vi "Main.vi"(11 "Module Admin":refnum<class "Delacor_lib_QMH_Module Admin.lvclass">) -> ()   [LabVIEW 2020, in "Settings.lvlib"]
doc: "This template is based off of the Queued Message Handler design pattern and the Queued Message Handler project template that ships with LabVIEW.\n\nThe main difference is that the queue is private to this module and communication between modules is performed via Broadcast and Request events.\n\nRequest events are wrapped in public API methods and are handled in the Event Handling Loop (EHL) of this VI. Any module can register for Broadcast events sent by this module. The EHL generates messages based on user interface actions.\n\nThe Message Handling Loop (MHL) processes messages generated by the EHL, or by other messages. The messages are string values, so new messages can be added easily to the Message Cases case structure in the MHL. Each message cluster can also provide an optional value for Message Data, which is a variant that can be converted to whatever message-specific data is required.\n_____\nBased on Delacor QMH Project Template 6.0.0.89."
uses:
  Settings.lvlib
  <vilib>/Delacor/Delacor QMH/Libraries/Module Admin_class/Delacor_lib_QMH_Module Admin.lvclass
  Acquisition/cluster analogico.ctl
  Acquisition/cluster digital.ctl
  Module Data--cluster.ctl
  Stop Argument--cluster.ctl
  <vilib>/Delacor/Delacor QMH/Libraries/Message Queue_class/Delacor_lib_QMH_Message Queue.lvclass/Delacor_lib_QMH_Message Queue.ctl
  <vilib>/Delacor/Delacor QMH/Libraries/Module Admin_class/Delacor_lib_QMH_Module Admin.lvclass/Delacor_lib_QMH_Module Admin.ctl
  ADD TASK Argument--cluster.ctl
  Erase all Argument--cluster.ctl
  <vilib>/Utility/miscctls.llb/LVPointTypeDef.ctl
  <vilib>/Delacor/Delacor QMH/Libraries/Message Queue_class/Delacor_lib_QMH_Enqueue Message (Single).vi
  <vilib>/Delacor/Delacor QMH/Libraries/Module Admin_class/Delacor_lib_QMH_Get External Launch.vi
  <vilib>/Utility/error.llb/Error Cluster From Error Code.vi
  <vilib>/ErrorRing/Error Ring.xnode
  <vilib>/Delacor/Delacor QMH/Libraries/Message Queue_class/Delacor_lib_QMH_Message Queue.lvclass
  Acquisition/CONTROLS.lvlib
panel:
  in  "EXIT":bool
  out "appended array":string[][](array[string])
  in  "NAME":string
  in  "RETURN":bool
  in  "ERASE":bool
  in  "ADD":bool
  in  "ANALOGICO/DIGITAL":bool
  in  "Adquisicion tiempo":i32
  in  "DAQ BOARD":tag
  in  "DIGITAL":T1={"Puertos Digital"=[], "Lineas Digital"=[], "Frecuencia Muestreo"=1000, "Puerto/Linea"=FALSE}
  in  "ANALOGICO":T2={"ANALOGICO CANALES"=[], "Numero de muestras"=1000, "Frecuencia de muestreo"=1000}
  out "error out":errorcluster
  out "Status":string
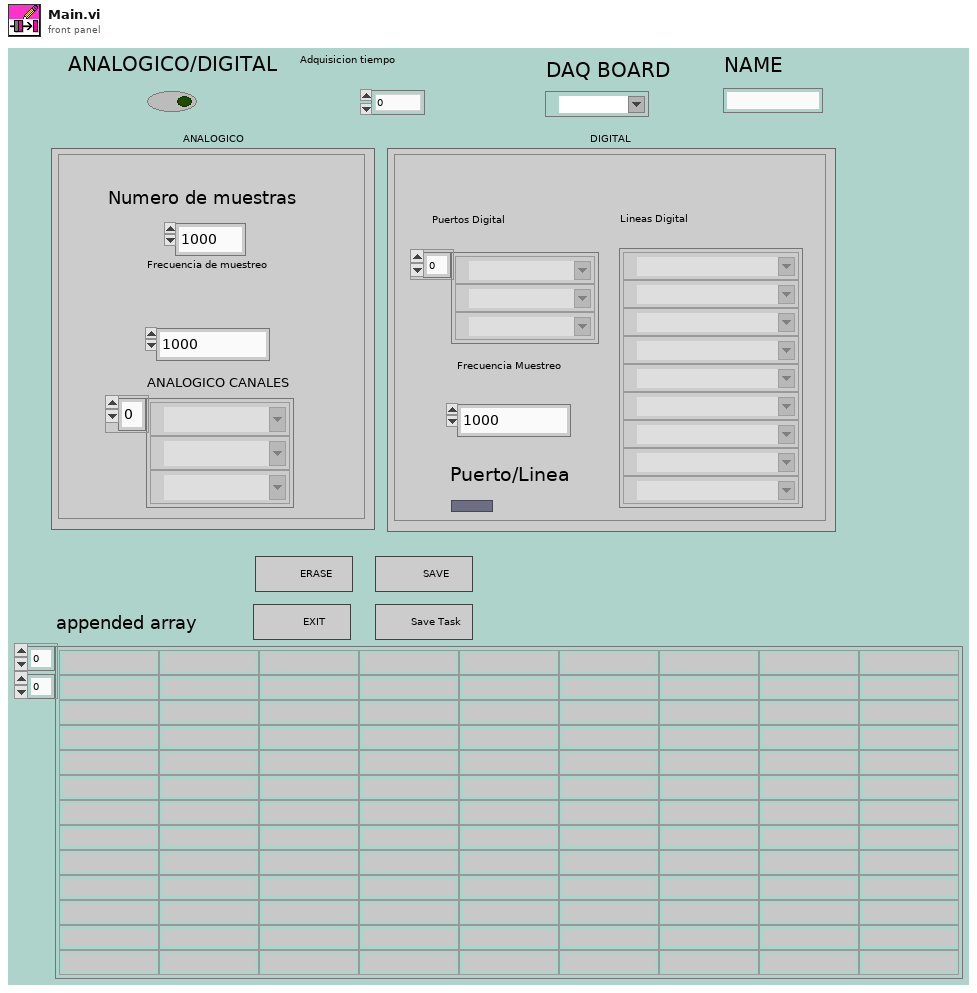
[diagram p1: front panel]
types:
  T1 = typedef "Acquisition.lvlib/CONTROLS.lvlib/cluster digital.ctl" = cluster{"Puertos Digital":tag[], "Lineas Digital":tag[], "Frecuencia Muestreo":u32, "Puerto/Linea":bool}
  T2 = typedef "Acquisition.lvlib/CONTROLS.lvlib/cluster analogico.ctl" = cluster{"ANALOGICO CANALES":tag[], "Numero de muestras":u32, "Frecuencia de muestreo":u32}
  T3 = typedef "Settings.lvlib/Request Events--cluster.ctl" = cluster{"Stop Module":refnum<user-event>, "Show Panel":refnum<user-event>, "Hide Panel":refnum<user-event>, "Get Module Execution Status":refnum<user-event>, "Show Diagram":refnum<user-event>, "ADD TASK":refnum<user-event>, "Erase all":refnum<user-event>}
  T4 = typedef "Settings.lvlib/Module Data--cluster.ctl" = cluster{"Status":string}
  T5 = enum32{"invalid lock state", "Not Locked", "Locked (No Password)", "Password-protected"}
  T6 = typedef "Settings.lvlib/Stop Argument--cluster.ctl" = cluster{"Origin":string, "Exit via Stop Module Req?":bool, "Wait for Module to stop?":bool}
  T7 = typedef "Settings.lvlib/ADD TASK Argument--cluster.ctl" = cluster{"ANALOGICO":T2, "DIGITAL":T1, "DAQ BOARD":tag, "Adquisicion tiempo":i32, "ANALOGICO/DIGITAL":bool}
  T8 = typedef "Settings.lvlib/Erase all Argument--cluster.ctl" = cluster{"Boolean":bool}
  T9 = typedef "LVPointTypeDef.ctl" = cluster{"Horizontal":i16, "Vertical":i16}
  T10 = enum32{"Invalid", "Standard", "Closed", "Hidden", "Minimized", "Maximized"}
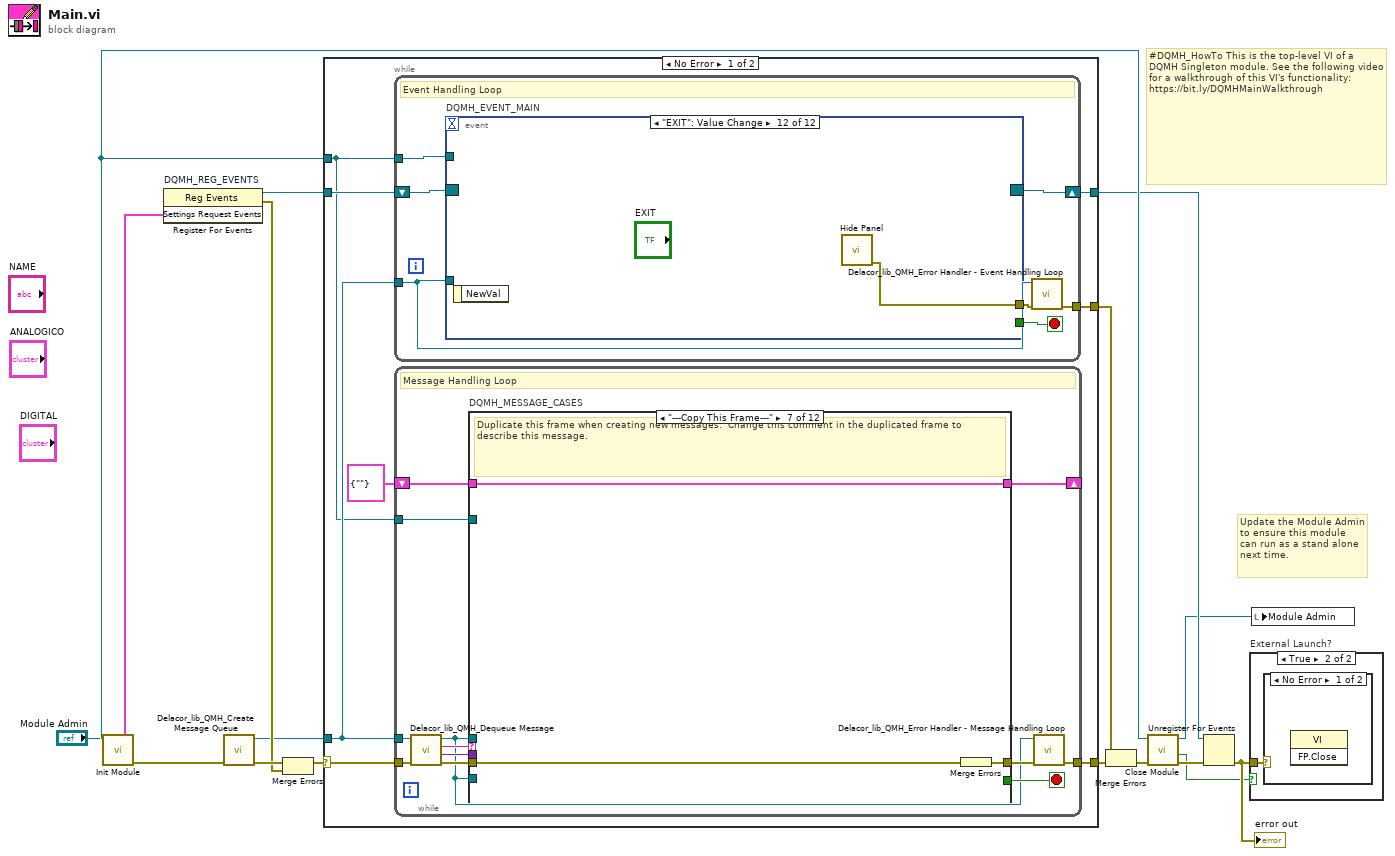
[diagram p0: block diagram]
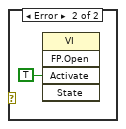
[diagram p3: hidden frame]
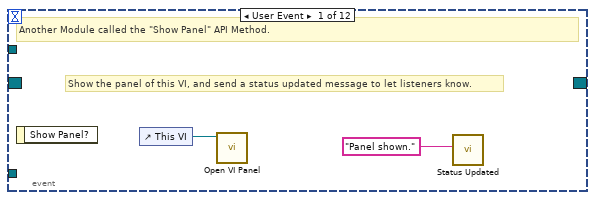
[diagram p4: hidden frame]
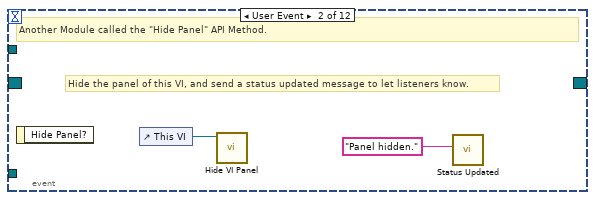
[diagram p5: hidden frame]
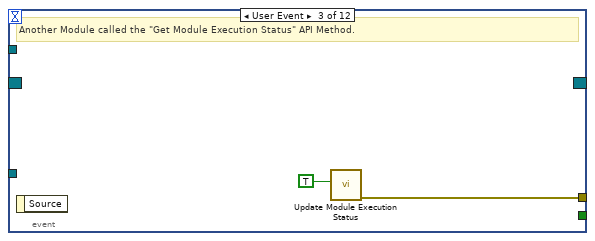
[diagram p6: hidden frame]
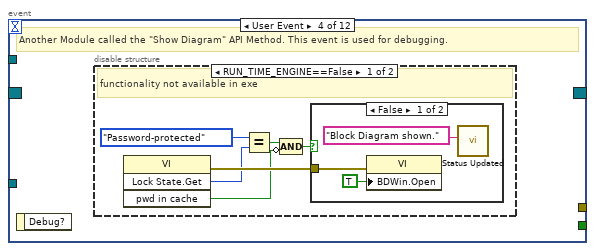
[diagram p7: hidden frame]
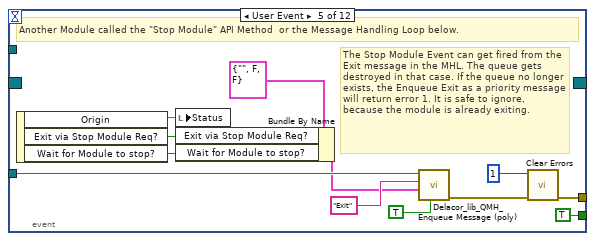
[diagram p10: hidden frame]
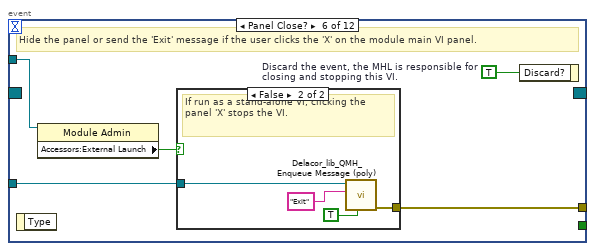
[diagram p11: hidden frame]
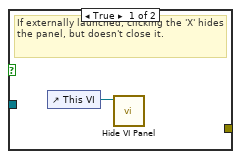
[diagram p12: hidden frame]
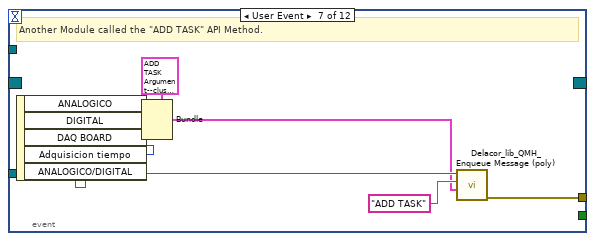
[diagram p13: hidden frame]
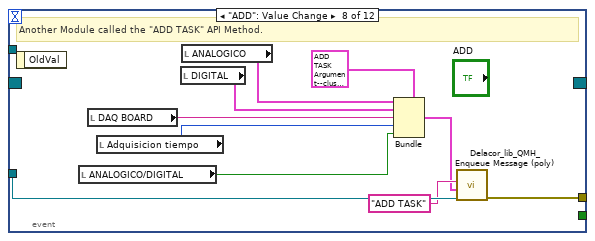
[diagram p14: hidden frame]
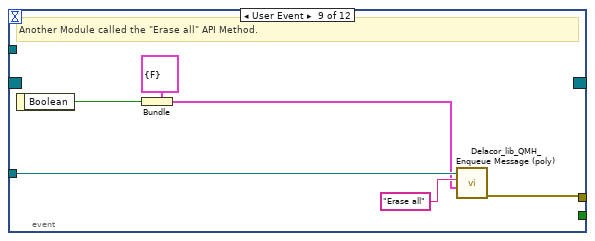
[diagram p15: hidden frame]
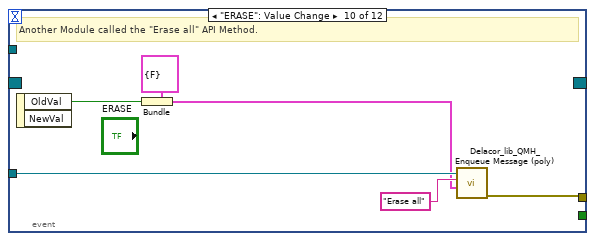
[diagram p16: hidden frame]
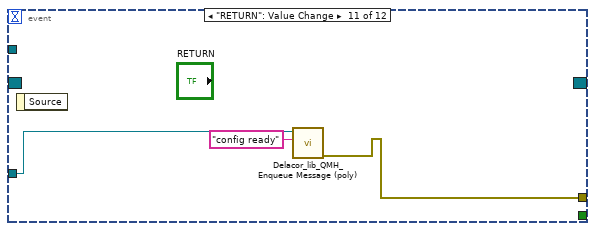
[diagram p17: hidden frame]
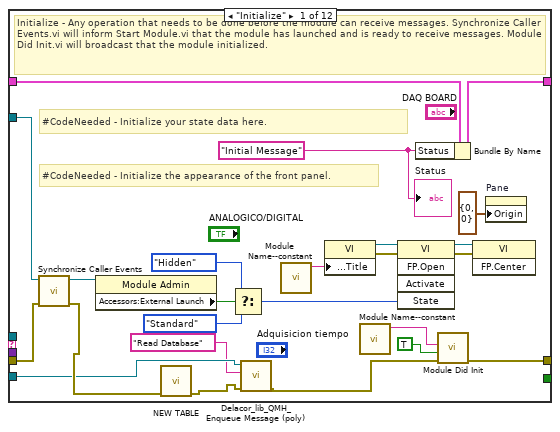
[diagram p18: hidden frame]
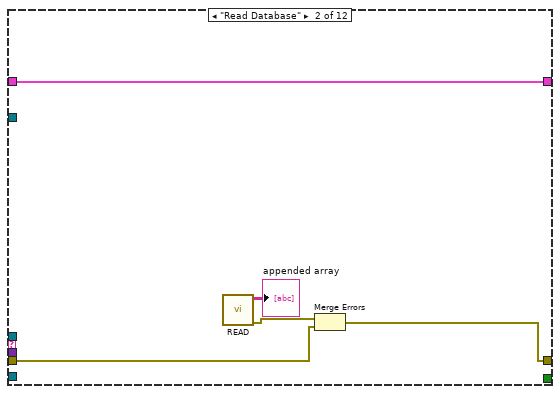
[diagram p19: hidden frame]
diagram:
  # "#DQMH_HowTo This is the top-level VI of a DQMH Singleton module. See the following video for a walkthrough of this VI's functionality: https://bit.ly/DQMHMainWalkthrough"
  # "Update the Module Admin to ensure this module can run as a stand alone next time."
  n1 = call "Init Module.vi"("Singleton Module Admin in"="Module Admin") -> ("error out"=w16:errorcluster, "Settings Request Events"=w5:T3, "Singleton Module Admin out"=w8:refnum<class "Delacor_lib_QMH_Module Admin.lvclass">)  [unwired: 8 in]
  n2 = register-events "DQMH_REG_EVENTS"(w5) -> (reference out=w6:refnum<event-registration>, error out=w9:errorcluster)  [unwired: 2 in]
  n3 = call <vilib>:"Delacor_lib_QMH_Create Message Queue.vi"("error in"=w16) -> ("error out"=w11:errorcluster, "Message Queue"=w4:refnum<class "Delacor_lib_QMH_Message Queue.lvclass">)  [unwired: 9 in]
  n4 = Merge Errors(w11, w9) -> (w10:errorcluster)
  n5 = case shown="No Error" w10 {
    selector: w10 -> [w23 w257]
    tunnel: [w25 w256] -> w17
    tunnel: [w22 w262] -> w7
    tunnel: w6 -> [w20 w262]
    tunnel: w4 -> [w19 w255]
    tunnel: [w24 _] -> w14
    tunnel: w8 -> [w18 w258]
    frame No Error {
      n6 = while {
        tunnel: w19 -> [w26]
        shift-right: [w29] -> w22
        shift-left: w20 -> [w30]
        tunnel: [w31] -> w24
        tunnel: w18 -> [w27]
        stop <- w28 stop-if-true
        # "Event Handling Loop"
        n7 = event "DQMH_EVENT_MAIN" shown="[11] \"EXIT\": Value Change" {
          selector: w30 -> [_ _ _ _ _ _ _ _ _ _ _ _]
          dyn-events: [_ _ _ _ _ _ _ _ _ _ _ _] -> w29
          timeout: _ -> [_ _ _ _ _ _ _ _ _ _ _ _]
          tunnel: [_ _ _ _ TRUE ("Discard?") _ _ _ _ _ _ _] -> w28
          tunnel: w26 -> [_ _ _ _ w55 w62 w79 w89 w95 w101 w103 _]
          tunnel: [_ _ w38 _ w58 w64 w70 w85 w90 w96 w104 w105] -> w32
          tunnel: w27 -> [_ _ _ _ _ w61 _ _ _ _ _ _]
          event User Event {
            # "Show the panel of this VI, and send a status updated message to let listeners know."
            # "Another Module called the \"Show Panel\" API Method."
            n8 = event-data() -> ()  [unwired: 1 in, 1 out]
            n9 = control-ref of="This VI"() -> (w34:refnum<vi>)
            n10 = call "Open VI Panel.vi"("VI"=w34) -> ()  [unwired: 10 in, 1 out]
            n11 = call "Status Updated.vi"("Status"="Panel shown." ("format string")) -> ()  [unwired: 10 in, 1 out]
          }
          event User Event {
            # "Hide the panel of this VI, and send a status updated message to let listeners know."
            # "Another Module called the \"Hide Panel\" API Method."
            n12 = event-data() -> ()  [unwired: 1 in, 1 out]
            n13 = control-ref of="This VI"() -> (w36:refnum<vi>)
            n14 = call "Hide VI Panel.vi"("VI"=w36) -> ()  [unwired: 10 in, 1 out]
            n15 = call "Status Updated.vi"("Status"="Panel hidden." ("format string")) -> ()  [unwired: 10 in, 1 out]
          }
          event User Event {
            # "Another Module called the \"Get Module Execution Status\" API Method."
            n16 = event-data() -> ()  [unwired: 1 in, 1 out]
            n17 = call "Update Module Execution Status.vi"("Running?"=TRUE) -> ("error out"=w38:errorcluster)  [unwired: 10 in]
          }
          event User Event {
            # "Another Module called the \"Show Diagram\" API Method. This event is used for debugging."
            n18 = event-data() -> ()  [unwired: 1 in, 1 out]
            n19 = disable-structure shown="RUN_TIME_ENGINE==False" {
              frame condition #0 (active) {
                # "functionality not available in exe"
                n20 = invoke class="VI" method="Lock State.Get"() -> (error out=w44:errorcluster, "Get Lock State"=w43:T5, "pwd in cache"=w40:bool)  [unwired: 4 in, 1 out]
                n21 = Equal?(x=T5."Password-protected", y=w43) -> (x = y?=w41:bool)
                n22 = Compound Arithmetic op=AND(w41, invert w40) -> (w39:bool)
                n23 = case shown="False" w39 {
                  tunnel: w44 -> [w47 _]
                  frame False {
                    n24 = property class="VI"(error in=w47, "BDWin.Open"=TRUE ("Block Diagram Window:Open")) -> ()  [unwired: 1 in, 2 out]
                    n25 = call "Status Updated.vi"("Status"="Block Diagram shown." ("format string")) -> ()  [unwired: 10 in, 1 out]
                  }
                  frame True {
                    # "Password-protected VI, and the password is not in the cache. Do not show the diagram."
                  }
                }
              }
              frame condition #1 {
              }
            }
          }
          event User Event {
            # "The Stop Module Event can get fired from the Exit message in the MHL. The queue gets destroyed in that case. If the queue no longer exists, the Enqueue Exit as a priority message will return error 1. It is safe to ignore, because the module is already exiting."
            # "Another Module called the \"Stop Module\" API Method  or the Message Handling Loop below."
            n26 = event-data() -> ("Origin"=w54:string, "Exit via Stop Module Req?"=w50:bool, "Wait for Module to stop?"=w49:bool)  [unwired: 1 in]
            n27 = local write "Status"(w54) -> ()
            n28 = Bundle By Name(cluster=T6 {"Origin"="", "Exit via Stop Module Req?"=FALSE, "Wait for Module to stop?"=FALSE} ("Stop Argument"), "Exit via Stop Module Req?"=w50, "Wait for Module to stop?"=w49) -> (w48:T6)
            n29 = call-poly <vilib>:"Delacor_lib_QMH_Enqueue Message (poly).vi"("Priority Message? (F)"=TRUE, "Message Data"=w48, "Message"="Exit", "Message Queue in"=w55) -> ("error out"=w59:errorcluster)  [unwired: 6 in, 1 out]
            n30 = call <vilib>:"Clear Errors.vi"("error in (no error)"=w59, "specific error code to clear (0: all)"=1) -> ("error out"=w58:errorcluster)  [unwired: 4 in, 1 out]
          }
          event Panel Close? {
            w63 = TRUE  # Discard the event, the MHL is responsible for closing and stopping this VI.
            # "Hide the panel or send the 'Exit' message if the user clicks the 'X' on the module main VI panel."
            n31 = event-data() -> ()  [unwired: 1 in, 1 out]
            n32 = property class="Module Admin"(reference=w61) -> ("Accessors:External Launch"=w60:bool)  [unwired: 1 in, 2 out]
            n33 = case shown="False" w60 {
              tunnel: w62 -> [_ w68]
              tunnel: [_ w69] -> w64
              frame True {
                # "If externally launched, clicking the 'X' hides the panel, but doesn't close it."
                n34 = control-ref of="This VI"() -> (w65:refnum<vi>)
                n35 = call "Hide VI Panel.vi"("VI"=w65) -> ()  [unwired: 10 in, 1 out]
              }
              frame False {
                # "If run as a stand-alone VI, clicking the panel 'X' stops the VI."
                n36 = call-poly <vilib>:"Delacor_lib_QMH_Enqueue Message (poly).vi"("Priority Message? (F)"=TRUE, "Message"="Exit", "Message Queue in"=w68) -> ("error out"=w69:errorcluster)  [unwired: 7 in, 1 out]
              }
            }
            n37 = event-data("Discard?"=w63) -> ()  [unwired: 1 in, 1 out]
          }
          event User Event {
            # "Another Module called the \"ADD TASK\" API Method."
            n38 = event-data() -> ("ANALOGICO"=w75:T2, "DIGITAL"=w74:T1, "DAQ BOARD"=w73:tag, "Adquisicion tiempo"=w72:i32, "ANALOGICO/DIGITAL"=w71:bool)  [unwired: 1 in]
            n39 = Bundle(cluster=T7 {"ANALOGICO"={"ANALOGICO CANALES"=[], "Numero de muestras"=1000, "Frecuencia de muestreo"=1000}, "DIGITAL"={"Puertos Digital"=[], "Lineas Digital"=[], "Frecuencia Muestreo"=1000, "Puerto/Linea"=FALSE}, "DAQ BOARD"="", "Adquisicion tiempo"=0, "ANALOGICO/DIGITAL"=FALSE} ("ADD TASK Argument"), "ANALOGICO"=w75, "DIGITAL"=w74, "DAQ BOARD"=w73, "Adquisicion tiempo"=w72, "ANALOGICO/DIGITAL"=w71) -> (w76:T7)
            n40 = call-poly <vilib>:"Delacor_lib_QMH_Enqueue Message (poly).vi"("Message Data"=w76, "Message"="ADD TASK", "Message Queue in"=w79) -> ("error out"=w70:errorcluster)  [unwired: 7 in, 1 out]
          }
          event "ADD": Value Change {
            # "Another Module called the \"ADD TASK\" API Method."
            n41 = event-data() -> ()  [unwired: 1 in, 1 out]
            n42 = local read "ANALOGICO/DIGITAL"() -> (w84:bool)
            n43 = local read "DAQ BOARD"() -> (w82:tag)
            n44 = local read "Adquisicion tiempo"() -> (w83:i32)
            n45 = local read "DIGITAL"() -> (w81:T1)
            n46 = local read "ANALOGICO"() -> (w80:T2)
            n47 = Bundle(cluster=T7 {"ANALOGICO"={"ANALOGICO CANALES"=[], "Numero de muestras"=1000, "Frecuencia de muestreo"=1000}, "DIGITAL"={"Puertos Digital"=[], "Lineas Digital"=[], "Frecuencia Muestreo"=1000, "Puerto/Linea"=FALSE}, "DAQ BOARD"="", "Adquisicion tiempo"=0, "ANALOGICO/DIGITAL"=FALSE} ("ADD TASK Argument"), "ANALOGICO"=w80, "DIGITAL"=w81, "DAQ BOARD"=w82, "Adquisicion tiempo"=w83, "ANALOGICO/DIGITAL"=w84) -> (w86:T7)
            n48 = call-poly <vilib>:"Delacor_lib_QMH_Enqueue Message (poly).vi"("Message Data"=w86, "Message"="ADD TASK", "Message Queue in"=w89) -> ("error out"=w85:errorcluster)  [unwired: 7 in, 1 out]
          }
          event User Event {
            # "Another Module called the \"Erase all\" API Method."
            n49 = event-data() -> ("Boolean"=w91:bool)  [unwired: 1 in]
            n50 = Bundle(cluster=T8 {"Boolean"=FALSE} ("Erase all Argument"), "Boolean"=w91) -> (w92:T8)
            n51 = call-poly <vilib>:"Delacor_lib_QMH_Enqueue Message (poly).vi"("Message Data"=w92, "Message"="Erase all", "Message Queue in"=w95) -> ("error out"=w90:errorcluster)  [unwired: 7 in, 1 out]
          }
          event "ERASE": Value Change {
            # "Another Module called the \"Erase all\" API Method."
            n52 = event-data() -> ("OldVal"=w97:bool)  [unwired: 1 in, 1 out]
            n53 = Bundle(cluster=T8 {"Boolean"=FALSE} ("Erase all Argument"), "Boolean"=w97) -> (w98:T8)
            n54 = call-poly <vilib>:"Delacor_lib_QMH_Enqueue Message (poly).vi"("Message Data"=w98, "Message"="Erase all", "Message Queue in"=w101) -> ("error out"=w96:errorcluster)  [unwired: 7 in, 1 out]
          }
          event "RETURN": Value Change {
            n55 = event-data() -> ()  [unwired: 1 in, 1 out]
            n56 = call-poly <vilib>:"Delacor_lib_QMH_Enqueue Message (poly).vi"("Message"="config ready", "Message Queue in"=w103) -> ("error out"=w104:errorcluster)  [unwired: 8 in, 1 out]
          }
          event "EXIT": Value Change {
            n57 = event-data() -> ()  [unwired: 1 in, 1 out]
            n58 = call "Hide Panel.vi"() -> ("error out"=w105:errorcluster)  [unwired: 11 in]
          }
        }
        n59 = call-dynamic "Delacor_lib_QMH_Error Handler - Event Handling Loop.vi"("error in"=w32, "Message Queue in"=w26) -> ("dup error in"=w31:errorcluster)  [unwired: 8 in, 1 out]
      }
      n60 = while {
        tunnel: w19 -> [w108]
        shift-right: [w112] -> _
        shift-left: T4 {"Status"=""} ("Data Cluster") -> [w113]
        tunnel: w23 -> [w116]
        tunnel: [w114] -> w25
        tunnel: w18 -> [w107]
        stop <- w111 stop-if-true
        # "Message Handling Loop"
        n61 = call-dynamic "Delacor_lib_QMH_Dequeue Message.vi"("error in"=w116, "Message Queue in"=w108) -> ("error out"=w115:errorcluster, "Message Data"=w109:variant, "Message"=w110:string, "Message Queue out"=w106:refnum<class "Delacor_lib_QMH_Message Queue.lvclass">)  [unwired: 6 in]
        n62 = case "DQMH_MESSAGE_CASES" shown="\"---Copy This Frame---\"" w110 {
          selector: w110 -> [_ _ _ _ _ _ _ _ _ _ _ w242]
          tunnel: w106 -> [_ _ _ w150 w176 _ _ _ _ w212 w234 _]
          tunnel: w115 -> [w139 w144 w148 w164 w183 w189 w195 w197 w202 w219 w240 w244]
          tunnel: [w138 w143 w148 w158 w177 w188 w194 w197 w201 w215 w237 w245] -> w117
          tunnel: w113 -> [w129 w146 w147 w163 w182 w192 w193 w196 w199 w214 w233 w243]
          tunnel: [w128 w146 w147 w163 w182 w192 w193 w196 w199 w214 w233 w243] -> w112
          tunnel: [_ _ _ _ _ _ _ _ _ _ w232 _] -> w111
          tunnel: w109 -> [_ _ _ w162 w181 _ _ _ _ w213 w231 _]
          tunnel: w107 -> [w130 _ _ _ _ _ _ _ _ w211 w226 _]
          tunnel: w106 -> [w119 _ _ _ _ _ _ _ _ _ _ _]
          frame "Initialize" {
            w124 = "Initial Message" ("Initial Message")
            # "#CodeNeeded - Initialize the appearance of the front panel."
            # "#CodeNeeded - Initialize your state data here."
            # "Initialize - Any operation that needs to be done before the module can receive messages. Synchronize Caller Events.vi will inform Start Module.vi that the module has launched and is ready to receive messages. Module Did Init.vi will broadcast that the module initialized."
            n63 = call "Synchronize Caller Events.vi"("error in (no error)"=w139, "Singleton Module Admin in"=w130) -> ("error out"=w122:errorcluster, "Singleton Module Admin out"=w125:refnum<class "Delacor_lib_QMH_Module Admin.lvclass">)  [unwired: 8 in]
            n64 = property class="Module Admin"(reference=w125) -> ("Accessors:External Launch"=w134:bool)  [unwired: 1 in, 2 out]
            n65 = call "NEW TABLE.vi"("error in (no error)"=w122) -> ("error out"=w121:errorcluster)  [unwired: 10 in]
            n66 = Select(t=T10."Hidden" ("State"), s=w134, f=T10."Standard" ("State")) -> (s? t:f=w131:T10)
            n67 = call-poly <vilib>:"Delacor_lib_QMH_Enqueue Message (poly).vi"("error in"=w121, "Message"="Read Database", "Message Queue in"=w119) -> ("error out"=w120:errorcluster)  [unwired: 7 in, 1 out]
            n68 = call "Module Name--constant.vi"() -> ("Module Name"=w137:string)  [unwired: 11 in]
            n69 = property class="VI"("Front Panel.Title"=w137) -> (reference out=w136:refnum<vi>, error out=w141:errorcluster)  [unwired: 2 in]
            n70 = call "Module Name--constant.vi"() -> ("Module Name"=w126:string)  [unwired: 11 in]
            n71 = invoke class="VI" method="FP.Open"(reference=w136, error in=w141, "State"=w131) -> (reference out=w135:refnum<vi>, error out=w140:errorcluster)  [unwired: 2 in, 3 out]
            n72 = Bundle By Name(cluster=w129, "Status"=w124) -> (w128:T4)
            n73 = call "Module Did Init.vi"("error in (no error)"=w120, "Initialized?"=TRUE, "Origin"=w126) -> ("error out"=w138:errorcluster)  [unwired: 8 in]
            n74 = invoke class="VI" method="FP.Center"(reference=w135, error in=w140) -> ()  [unwired: 1 in, 3 out]
            n75 = property on="Pane" class="Pane"("Origin"=T9 {"Horizontal"=0, "Vertical"=0}) -> ()  [unwired: 2 in, 2 out]
            "Status" <- w124
          }
          frame "Read Database" {
            n76 = call "READ.vi"() -> ("error out"=w145:errorcluster, "appended array"=→"appended array":string[][])  [unwired: 9 in, 1 out]
            n77 = Merge Errors(w145, w144) -> (w143:errorcluster)
          }
          frame "---Module Specific---" {
            # "Separator -- The following cases handle messages specific to this Module."
          }
          frame "ADD TASK" {
            # "AGREGA EL TASK"
            n78 = Variant To Data(error in=w164, type=T7 {"ANALOGICO"={"ANALOGICO CANALES"=[], "Numero de muestras"=1000, "Frecuencia de muestreo"=1000}, "DIGITAL"={"Puertos Digital"=[], "Lineas Digital"=[], "Frecuencia Muestreo"=1000, "Puerto/Linea"=FALSE}, "DAQ BOARD"="", "Adquisicion tiempo"=0, "ANALOGICO/DIGITAL"=FALSE} ("ADD TASK Argument"), Variant=w162) -> (data=w160:T7, error out=w151:errorcluster)
            n79 = Unbundle By Name(w160) -> ("ANALOGICO"=w156:T2, "DIGITAL"=w155:T1, "DAQ BOARD"=w153:tag, "Adquisicion tiempo"=w154:i32, "ANALOGICO/DIGITAL"=w157:bool)
            n80 = call-poly <vilib>:"Delacor_lib_QMH_Enqueue Message (poly).vi"("error in"=w151, "Message"="Read Database", "Message Queue in"=w150) -> ("error out"=w152:errorcluster)  [unwired: 7 in, 1 out]
            n81 = case shown="False" w157 {
              tunnel: [w168 w172] -> w159
              tunnel: w156 -> [w167 _]
              tunnel: w155 -> [_ w171]
              tunnel: w154 -> [w166 w170]
              tunnel: w153 -> [w165 w169]
              frame False {
                n82 = call "UPDATE.vi"("DAQ BOARD"=w165, "Adquisicion tiempo"=w166, "ANALOGICO"=w167) -> ("error out"=w168:errorcluster)  [unwired: 8 in]
              }
              frame True {
                n83 = call "UPDATE.vi"("DAQ BOARD"=w169, "Adquisicion tiempo"=w170, "DIGITAL"=w171) -> ("error out"=w172:errorcluster)  [unwired: 8 in]
              }
            }
            n84 = Merge Errors(w159, w152) -> (w158:errorcluster)
          }
          frame "Erase all" {
            # "Borra todo de la base de datos"
            n85 = Variant To Data(error in=w183, type=T8 {"Boolean"=FALSE} ("Erase all Argument"), Variant=w181) -> (data=w179:T8, error out=w174:errorcluster)
            n86 = Unbundle By Name(w179) -> ()  [unwired: 1 out]
            n87 = call-poly <vilib>:"Delacor_lib_QMH_Enqueue Message (poly).vi"("error in"=w174, "Message"="Read Database", "Message Queue in"=w176) -> ("error out"=w173:errorcluster)  [unwired: 7 in, 1 out]
            n88 = call "erase.vi"() -> ("error out"=w178:errorcluster)  [unwired: 11 in]
            n89 = Merge Errors(w178, w173) -> (w177:errorcluster)
          }
          frame "config ready" {
            n90 = local read "NAME"() -> (w185:string)
            n91 = call "READ.vi"() -> ("error out"=w190:errorcluster, "Result Set"=w191:string[][])  [unwired: 9 in, 1 out]
            n92 = call "Nombre task.vi"("NAME"=w185) -> ("error out"=w184:errorcluster)  [unwired: 10 in]
            n93 = call "Task to do.vi"("error in"=w190, "Result Set"=w191) -> ("error out"=w187:errorcluster)  [unwired: 9 in]
            n94 = call "Hide Panel.vi"("error in (no error)"=w187) -> ("error out"=w186:errorcluster)  [unwired: 10 in]
            n95 = Merge Errors(w186, w189, w184) -> (w188:errorcluster)
          }
          frame "---Copy This Frame---" {
            # "Duplicate this frame when creating new messages.  Change this comment in the duplicated frame to describe this message."
            n96 = Merge Errors(w195) -> (w194:errorcluster)
          }
          frame "---Exit and Error Handling---" {
            # "Separator - The following cases handle errors and exit messages."
          }
          frame "Simulate MHL Error" {
            # "#DQMH_HowTo The 'Simulate MHL Error' button  illustrates how the MHL handles errors. This event is instructional in nature and can be removed."
            # "Simulate an error occurring at the MHL"
            n97 = call "Module Name--constant.vi"() -> ("Module Name"=w198:string)  [unwired: 11 in]
            n98 = xnode "Error Ring"("parameter 0"=w198) -> ("error out"=w200:errorcluster)
            n99 = Merge Errors(w202, w200) -> (w201:errorcluster)
          }
          frame "Error" {
            # "#CodeRecommended - If you ever change the name of this \"Error\" message, you'll need to update the name in the Check Loop Error.vi as well."
            # "#CodeRecommended - If the module is running in standalone mode (External Launch = FALSE), this code will pop up an error dialog and call the 'Exit' message if an error occurs. Add more fine-grained error handling here."
            # "Error - Check the error message data and respond accordingly. This message is sent by the \"Error Handler\" VIs at the end of each loop in this application."
            n100 = property class="Module Admin"(reference=w211) -> ("Accessors:External Launch"=w210:bool)  [unwired: 1 in, 2 out]
            n101 = Variant To Data(error in=w219, type=errorcluster {"status"=FALSE, "code"=0, "source"=""} ("error constant"), Variant=w213) -> (data=w220:errorcluster, error out=w217:errorcluster)
            n102 = call "Error Reported.vi"("Error"=w220) -> ()  [unwired: 10 in, 1 out]
            n103 = case shown="False" w210 {
              tunnel: [w225 _] -> w216
              tunnel: w212 -> [w223 _]
              tunnel: w220 -> [w224 _]
              frame False {
                # "If the module is running standalone, then pop up an error dialog and call the \"Exit\" message."
                n104 = call <vilib>:"Simple Error Handler.vi"("error in (no error)"=w224) -> ()  [unwired: 4 in, 5 out]
                n105 = call-poly <vilib>:"Delacor_lib_QMH_Enqueue Message (poly).vi"("Priority Message? (F)"=TRUE, "Message"="Exit", "Message Queue in"=w223) -> ("error out"=w225:errorcluster)  [unwired: 7 in, 1 out]
              }
              frame True {
                # "If the module was launched externally, calling the Error Reported broadcast VI is the only action performed by the \"Error\" message. The module's caller can then process the error appropriately."
              }
            }
            n106 = Merge Errors(w217, w216) -> (w215:errorcluster)
            n107 = local write "error out"(w215) -> ()
          }
          frame "Exit" {
            w230 = 91  # 91: not all Exit messages will have an argument
            w232 = TRUE  # Stop the VI
            # "Release the message queue reference"
            # "#CodeNeeded - Add any required cleanup code here"
            # "Exit - Exit the application."
            n108 = Variant To Data(error in=w240, type=T6 {"Origin"="", "Exit via Stop Module Req?"=FALSE, "Wait for Module to stop?"=FALSE} ("Stop Argument"), Variant=w231) -> (data=w228:T6, error out=w236:errorcluster)
            n109 = call <vilib>:"Clear Errors.vi"("error in (no error)"=w236, "specific error code to clear (0: all)"=w230) -> ("error out"=w239:errorcluster)  [unwired: 4 in, 1 out]
            n110 = control-ref of="This VI"() -> (w227:refnum<vi>)
            n111 = call-dynamic "Delacor_lib_QMH_Release Message Queue.vi"("error in"=w239, "Message Queue"=w234) -> ("error out"=w238:errorcluster)  [unwired: 9 in]
            n112 = call "Handle Exit.vi"("Stop Argument"=w228, "Admin in"=w226, "VI reference"=w227) -> ("error out"=w235:errorcluster)  [unwired: 7 in, 1 out]
            n113 = Merge Errors(w238, w235) -> (w237:errorcluster)
          }
          frame Default {
            # "'Default' case only runs if there is a message that isn't defined in any of the other cases.  Output a programming error."
            n114 = call "Module Name--constant.vi"() -> ("Module Name"=w241:string)  [unwired: 11 in]
            n115 = xnode "Error Ring"("parameter 0"=w242, "parameter 1"=w241) -> ("error out"=w246:errorcluster)
            n116 = Merge Errors(w244, w246) -> (w245:errorcluster)
          }
        }
        n117 = call-dynamic "Delacor_lib_QMH_Error Handler - Message Handling Loop.vi"("error in"=w117, "Message Queue in"=w106) -> ("dup error in"=w114:errorcluster)  [unwired: 8 in, 1 out]
      }
    }
    frame Error {
      # "Synchronize Caller Events.vi will inform Start Module.vi that the module has launched and will let the code calling Start Module.vi register for broadcasts and would permit the caller receive the broadcast that an error occurred at launch time."
      n118 = call-dynamic "Delacor_lib_QMH_Release Message Queue.vi"("error in"=w257, "Message Queue"=w255) -> ("error out"=w256:errorcluster)  [unwired: 9 in]
      n119 = call "Synchronize Caller Events.vi"("Singleton Module Admin in"=w258) -> ("error out"=w263:errorcluster)  [unwired: 9 in, 1 out]
      n120 = call "Module Name--constant.vi"() -> ("Module Name"=w261:string)  [unwired: 11 in]
      n121 = Format Into String(format string="An error occurred during initialization. %s is no longer running.", w261) -> (resulting string=w259:string)  [unwired: 2 in, 1 out]
      n122 = Merge Errors(w256, w263) -> (w264:errorcluster)
      n123 = call "Error Reported.vi"("Additional Information"=w259, "Error"=w264) -> ()  [unwired: 9 in, 1 out]
    }
  }
  n124 = Merge Errors(w14, w17) -> (w13:errorcluster)
  n125 = call "Close Module.vi"("error in (no error)"=w13, "Module Admin in"=w8) -> ("error out"=w15:errorcluster, "External Launch"=w1:bool, "Module Admin out"=w2:refnum<class "Delacor_lib_QMH_Module Admin.lvclass">)  [unwired: 7 in]
  n126 = Unregister For Events(event registration refnum=w7, error in=w15) -> (error out=w12:errorcluster)
  "error out" <- w12
  n127 = case "External Launch?" shown="True" w1 {
    tunnel: w12 -> [_ w265]
    frame False {
    }
    frame True {
      n128 = case shown="No Error" w265 {
        frame No Error {
          n129 = invoke class="VI" method="FP.Close"() -> ()  [unwired: 3 in, 3 out]
        }
        frame Error {
          n130 = invoke class="VI" method="FP.Open"("Activate"=TRUE ("Activate?")) -> ()  [unwired: 4 in, 5 out]
        }
      }
    }
  }
  n131 = local write "Module Admin"(w2) -> ()
